vi "queryT7Inclinometer.vi"(8 "error in (no error)":errorcluster, 11 "Model in":refnum<class "Model.lvclass">) -> (0 "error out":errorcluster, 3 "Model out":refnum<class "Model.lvclass">)   [LabVIEW 2016, in "Model.lvclass"]
uses:
  Model.lvclass
  Model.lvclass/Model.ctl
  Resources/FPGA/FPGA.lvclass
  Common_RT_T7Inclinometer/T7Inclinometer/T7Inclinometer.lvclass
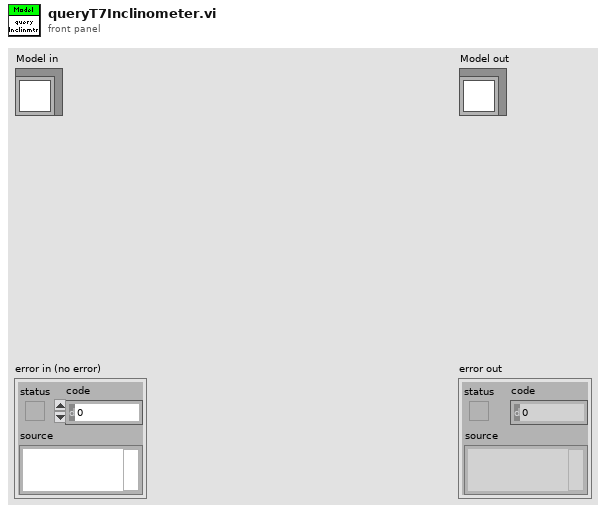
[diagram p1: front panel]
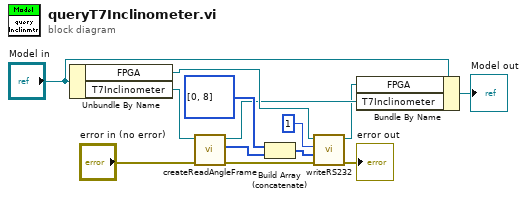
[diagram p0: block diagram]
diagram:
  n1 = Unbundle By Name("Model in") -> ("FPGA"=w13:refnum<class "FPGA.lvclass">, "T7Inclinometer"=w11:refnum<class "T7Inclinometer.lvclass">)
  n2 = call "createReadAngleFrame.vi"("error in (no error)"="error in (no error)", "T7Inclinometer in"=w11) -> ("error out"=w6:errorcluster, "Message"=w10:u8[], "T7Inclinometer out"=w3:refnum<class "T7Inclinometer.lvclass">)  [unwired: 7 in]
  n3 = Build Array (concatenate)(u8[] [0, 8] ("element"), w10) -> (w8:u8[])
  n4 = call "writeRS232.vi"("error in (no error)"=w6, "Data"=w8, "Port"=u8 1, "FPGA in"=w13) -> ("error out"=→"error out":errorcluster, "FPGA out"=w2:refnum<class "FPGA.lvclass">)  [unwired: 6 in]
  n5 = Bundle By Name(cluster="Model in", "FPGA"=w2, "T7Inclinometer"=w3) -> (→"Model out":refnum<class "Model.lvclass">)
